vi "Save doc pdf.vi"(8 "error in (no error)":errorcluster, 9 "File Name":string, 10 "DesignRequest":T1, 11 "ActiveDocument":refnum<k7>) -> (0 "error out":errorcluster)   [LabVIEW 2012, in "Design Server.lvlib"]
uses:
  Design Server.lvlib
  Design Request.ctl
  Variable cluster.ctl
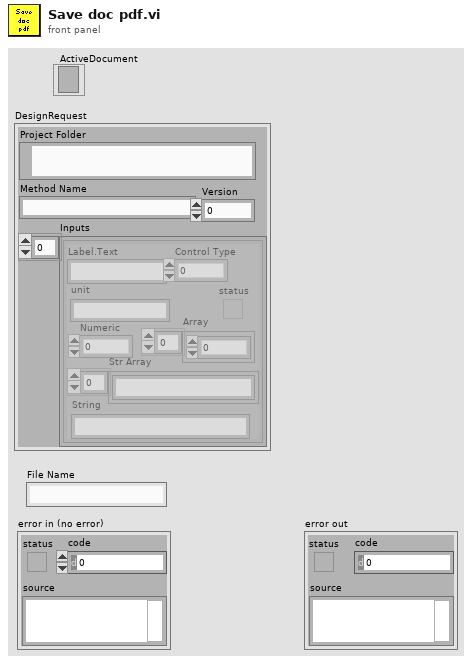
[diagram p1: front panel]
types:
  T1 = typedef "Design Server.lvlib/Design Request.ctl" = cluster{"Project Folder":path, "Method Name":string, "Inputs":T2, "Version":i32}
  T2 = typedef "Design Server.lvlib/Variable cluster.ctl" = cluster{"Label.Text":string, "Control Type":u32, "Numeric":dbl, "Array":dbl[], "status":bool, "Str Array":string[], "String":string, "unit":string}[]
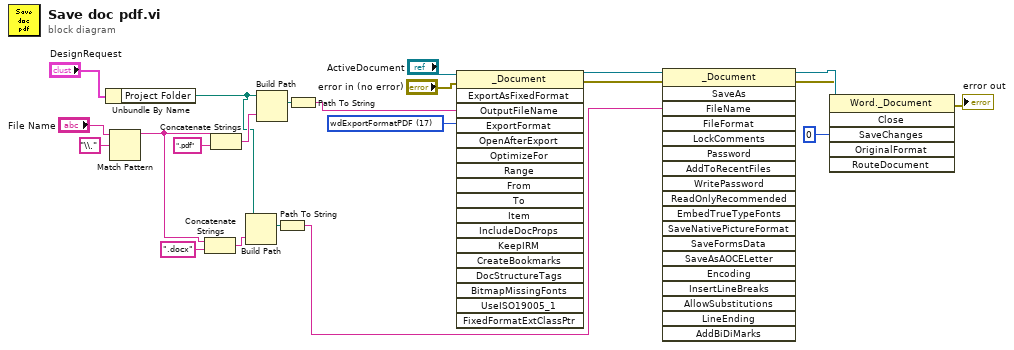
[diagram p0: block diagram]
diagram:
  w16 = 17 items=["wdExportFormatPDF"=17, "wdExportFormatXPS"=18] ("ExportFormat")
  n1 = Unbundle By Name("DesignRequest") -> ("Project Folder"=w2:path)
  n2 = Match Pattern(string="File Name", regular expression="\\.") -> (before substring=w5:string)  [unwired: 1 in, 3 out]
  n3 = Concatenate Strings(w5, ".docx" ("string")) -> (w3:string)
  n4 = Concatenate Strings(w5, ".pdf" ("string")) -> (w9:string)
  n5 = Build Path(base path=w2, name or relative path=w3) -> (appended path=w4:path)
  n6 = Build Path(base path=w2, name or relative path=w9) -> (appended path=w8:path)
  n7 = Path To String(path=w4) -> (string=w1:string)
  n8 = Path To String(path=w8) -> (string=w7:string)
  n9 = invoke class="_Document" method="ExportAsFixedFormat"(reference="ActiveDocument", error in="error in (no error)", "OutputFileName"=w7, "ExportFormat"=w16) -> (reference out=w21:refnum<k7>, error out=w19:errorcluster)  [unwired: 14 in, 16 out]
  n10 = invoke class="_Document" method="SaveAs"(reference=w21, error in=w19, "FileName"=w1) -> (reference out=w22:refnum<k7>, error out=w20:errorcluster)  [unwired: 16 in, 17 out]
  n11 = invoke class="Word._Document" method="Close"(reference=w22, error in=w20, "SaveChanges"=0) -> (error out=→"error out":errorcluster)  [unwired: 3 in, 5 out]
